vi "Upshift.vi"(11 "Cluster":T1) -> (3 "Upshift?":bool)   [LabVIEW 2013]
uses:
  Drive Train Metrics.ctl
  CmdFlag.ctl
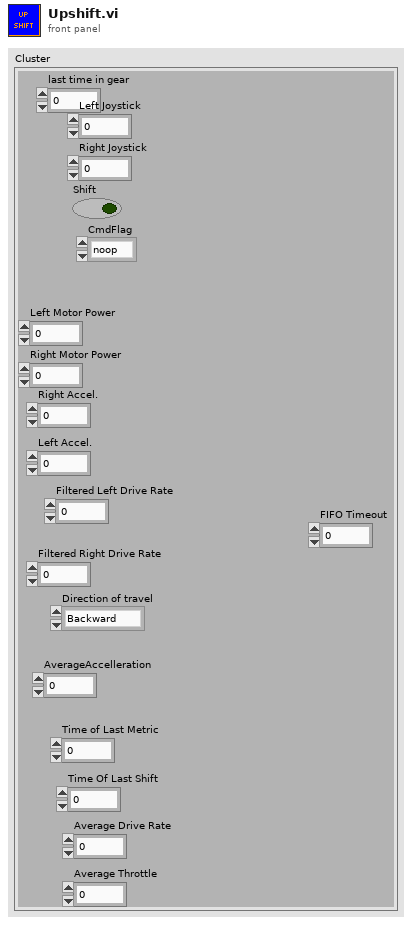
[diagram p1: front panel]
types:
  T1 = typedef "Drive Train Metrics.ctl" = cluster{"last time in gear":u32, "Shift":bool, "Right Joystick":dbl, "Left Joystick":dbl, "CmdFlag":T2, "Right Motor Power":dbl, "Left Motor Power":dbl, "Right Accel.":dbl, "Left Accel.":dbl, "Filtered Left Drive Rate":dbl, "Filtered Right Drive Rate":dbl, "Direction of travel":enum16{"Backward", "Forward", "Spin"}, "AverageAccelleration":dbl, "Time of Last Metric":u32, "Time Of Last Shift":dbl, "Average Drive Rate":dbl, "Average Throttle":dbl, "FIFO Timeout":i32}
  T2 = typedef "CmdFlag.ctl" = enum16{"noop", "suspend", "resume"}
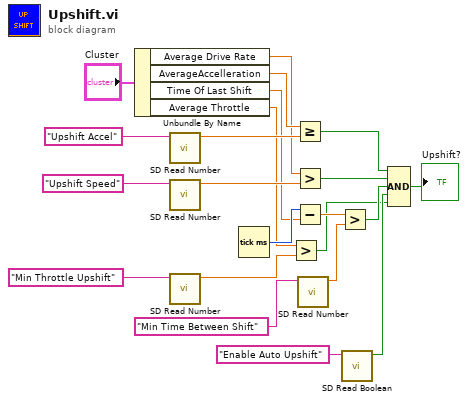
[diagram p0: block diagram]
diagram:
  n1 = Unbundle By Name("Cluster") -> ("Average Drive Rate"=w11:dbl, "AverageAccelleration"=w17:dbl, "Time Of Last Shift"=w15:dbl, "Average Throttle"=w4:dbl)
  n2 = call <vilib>:"SD Read Number.vi"("Name"="Upshift Accel") -> ("Numeric"=w21:dbl)  [unwired: 8 in, 2 out]
  n3 = call <vilib>:"SD Read Number.vi"("Name"="Upshift Speed") -> ("Numeric"=w22:dbl)  [unwired: 8 in, 2 out]
  n4 = call <vilib>:"SD Read Number.vi"("Name"="Min Throttle Upshift") -> ("Numeric"=w2:dbl)  [unwired: 8 in, 2 out]
  n5 = Tick Count (ms)() -> (millisecond timer value=w16:u32)
  n6 = Greater?(x=w4, y=w2) -> (0:w1:bool)
  n7 = Greater Or Equal?(x=w17, y=w21) -> (x >= y?=w9:bool)
  n8 = Greater?(x=w11, y=w22) -> (0:w10:bool)
  n9 = Subtract(x=w16, y=w15) -> (x-y=w14:dbl)
  n10 = call <vilib>:"SD Read Number.vi"("Name"="Min Time Between Shift") -> ("Numeric"=w13:dbl)  [unwired: 8 in, 2 out]
  n11 = Greater?(x=w14, y=w13) -> (0:w8:bool)
  n12 = call <vilib>:"SD Read Boolean.vi"("Name"="Enable Auto Upshift") -> ("Boolean"=w5:bool)  [unwired: 8 in, 2 out]
  n13 = Compound Arithmetic op=AND(w9, w10, w8, w5, w1) -> (→"Upshift?":bool)
